vi "Upload Score.vi"(7 "submission":i32, 8 "error in (no error)":errorcluster, 9 "result":string, 10 "status":string, 11 "Run Time":dbl) -> (0 "error out":errorcluster, 2 "Response":string, 5 "Profile URL":string)   [LabVIEW 2024, in "Wordle Scorer.lvlib"]
uses:
  Wordle Scorer.lvlib
  Score Post.ctl
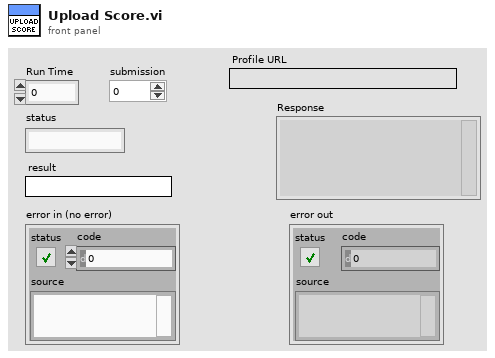
[diagram p1: front panel]
types:
  T1 = typedef "Wordle Scorer.lvlib/Score Post.ctl" = cluster{"scorer":string, "key":string, "submission":i32, "score":dbl, "status":string, "result":string}
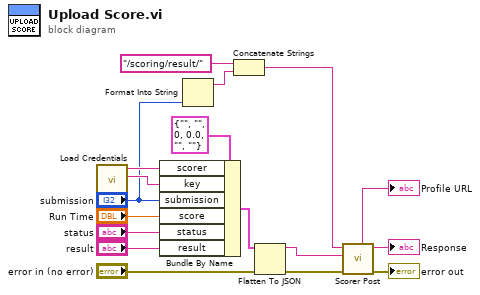
[diagram p0: block diagram]
diagram:
  n1 = call "Load Credentials.vi"() -> ("Key"=w11:string, "ID"=w12:string)  [unwired: 9 in, 1 out]
  n2 = Bundle By Name(cluster=T1 {"scorer"="", "key"="", "submission"=0, "score"=0.0, "status"="", "result"=""} ("Score Upload"), "scorer"=w12, "key"=w11, "submission"="submission", "score"="Run Time", "status"="status", "result"="result") -> (w10:T1)
  n3 = Format Into String("submission") -> (resulting string=w2:string)  [unwired: 3 in, 1 out]
  n4 = Concatenate Strings("/scoring/result/" ("Path"), w2) -> (w3:string)
  n5 = Flatten To JSON(anything=w10, error in (no error)="error in (no error)") -> (JSON string=w7:string, 11:w8:errorcluster)  [unwired: 1 in]
  n6 = call "Scorer Post.vi"("error in (no error)"=w8, "buffer"=w7, "Path"=w3) -> ("error out"=→"error out":errorcluster, "Content"=→"Response":string, "Profile URL"=→"Profile URL":string)  [unwired: 5 in, 1 out]
